vi "Signal-error.vi"(8 "error in (no error)":errorcluster, 11 "ModComm in":T1) -> (0 "error out":errorcluster, 3 "ModComm out":T1)   [LabVIEW 2013, in "Server.lvlib" / "Server.lvclass"]
uses:
  Server.lvclass
  Object-reference.ctl
  Server.lvclass/Server.ctl
  Read Error log.vi
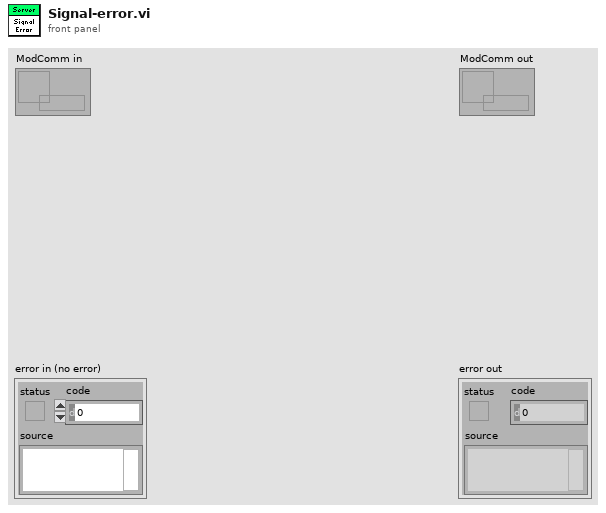
[diagram p1: front panel]
types:
  T1 = typedef "Server.lvlib/Server.lvclass/Object-reference.ctl" = refnum<data-value>
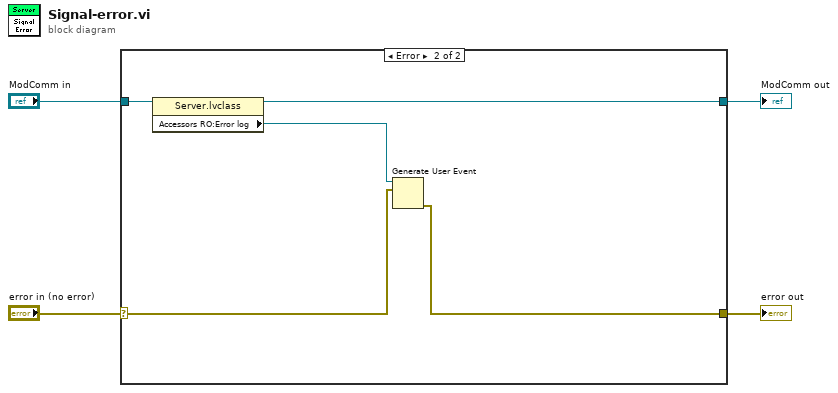
[diagram p0: block diagram]
diagram:
  n1 = case shown="Error" "error in (no error)" {
    selector: "error in (no error)" -> [w6 w8]
    tunnel: "ModComm in" -> [w5 w11]
    tunnel: [w5 w10] -> w3
    tunnel: [w6 w7] -> w2
    frame No Error {
    }
    frame Error {
      n2 = property class="Server.lvclass"(reference=w11) -> (reference out=w10:T1, "Accessors RO:Error log"=w9:refnum<user-event>)  [unwired: 1 in, 1 out]
      n3 = Generate User Event(user event=w9, event data cluster=w8) -> (error out=w7:errorcluster)  [unwired: 2 in, 1 out]
    }
  }
  "error out" <- w2
  "ModComm out" <- w3
